vi "Log Info.vi"(4 "Message":string) -> (1 "error out":errorcluster)   [LabVIEW 2015]
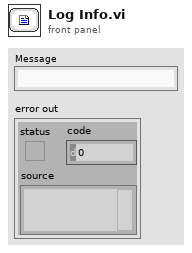
[diagram p1: front panel]
types:
  T1 = cluster{"Log Level":enum16{"INFO", "DEBUG", "WARN", "ERROR"}, "Time Stamp":timestamp, "Call Chain":string[], "Message":string}
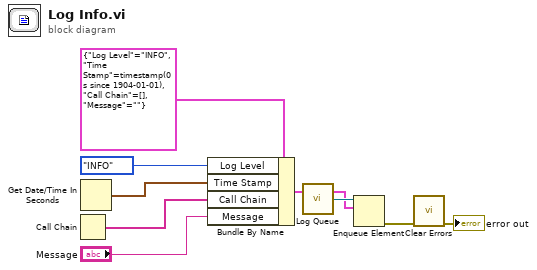
[diagram p0: block diagram]
diagram:
  n1 = Call Chain() -> (call chain=w4:string[])
  n2 = Get Date/Time In Seconds() -> (seconds since 1Jan1904=w5:timestamp)
  n3 = Bundle By Name(cluster=T1 {"Log Level"=enum."INFO", "Time Stamp"=timestamp(0 s since 1904-01-01), "Call Chain"=[], "Message"=""} ("element"), "Log Level"=enum16{"INFO", "DEBUG", "WARN", "ERROR"}."INFO", "Time Stamp"=w5, "Call Chain"=w4, "Message"="Message") -> (w7:T1)
  n4 = call "Log Queue.vi"() -> ("Log Queue"=w9:refnum<queue>)  [unwired: 5 in]
  n5 = Enqueue Element(queue=w9, element=w7) -> (error out=w2:errorcluster)  [unwired: 2 in, 2 out]
  n6 = call <vilib>:"Clear Errors.vi"("error in (no error)"=w2) -> ("error out"=→"error out":errorcluster)  [unwired: 5 in, 1 out]
